vi "Read Capacitor.vi"(0 "Arduino Resource in":T3, 5 "Analog input Pin":u8, 9 "Resistor Pin":u8, 11 "error in":errorcluster) -> (4 "Arduino Resource out":T3, 8 "Time (us)":string, 15 "error out":errorcluster)   [LabVIEW 2015]
doc: "Writes the specified value on the selected digital output pin (D0 - D13). The pin must fist be configured as an output using the Arduino Set Digital Pin Mode VI."
uses:
  <vilib>/LabVIEW Interface for Arduino/Type Defs/Board Type.ctl
  <vilib>/LabVIEW Interface for Arduino/Type Defs/Connection Type.ctl
  <vilib>/LabVIEW Interface for Arduino/LabVIEW Interface for Arduino.lvlib
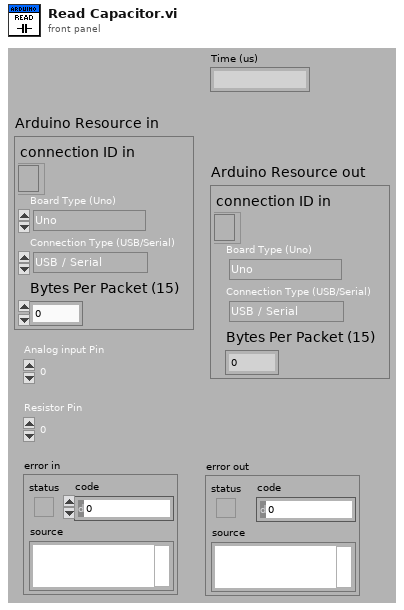
[diagram p1: front panel]
types:
  T1 = typedef "LabVIEW Interface for Arduino.lvlib/Board Type.ctl" = enum16{"Uno", "Dimuelanove w/Atmega 328", "Mega 2560"}
  T2 = typedef "LabVIEW Interface for Arduino.lvlib/Connection Type.ctl" = enum8{"USB / Serial", "XBEE", "BlueSmirf (Bluetooth)"}
  T3 = cluster{"connection ID in":refnum<k31>, "Board Type (Uno)":T1, "Connection Type (USB/Serial)":T2, "Bytes Per Packet (15)":u32}
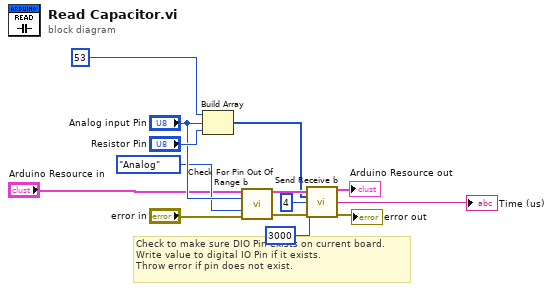
[diagram p0: block diagram]
diagram:
  # "Check to make sure DIO Pin exists on current board.\nWrite value to digital IO Pin if it exists.\nThrow error if pin does not exist."
  n1 = Build Array(53, "Analog input Pin", "Resistor Pin") -> (w7:i32[])
  n2 = call "Check For Pin Out Of Range b.vi"("Arduino Resource in"="Arduino Resource in", "User Pin Number"="Analog input Pin", "Pin Type"=enum16{"Analog", "Digital"}."Analog", "error in"="error in") -> ("Arduino Resource out"=w10:T3, "error out"=w8:errorcluster)  [unwired: 10 in]
  n3 = call "Send Receive b.vi"("Arduino Resource"=w10, "Data"=w7, "Bytes To Read (0)"=u32 4, "Time Out (100 ms)"=3000, "error in"=w8) -> ("Arduino Resource out"=→"Arduino Resource out":T3, "Read Buffer"=→"Time (us)":string, "error out"=→"error out":errorcluster)  [unwired: 8 in]
